vi "TEST - Convert Dirs to VI Libraries (proxy).vi"(8 "error in (no error)":errorcluster) -> (0 "error out":errorcluster, 2 "pass":bool)   [LabVIEW 2020]
uses:
  <userlib>/_OpenG.lib/error/error.llb/openg_error.lvlib
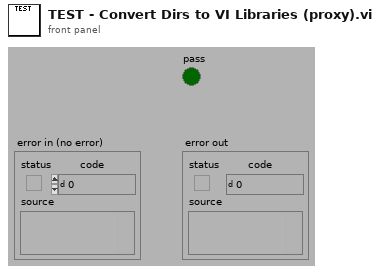
[diagram p1: front panel]
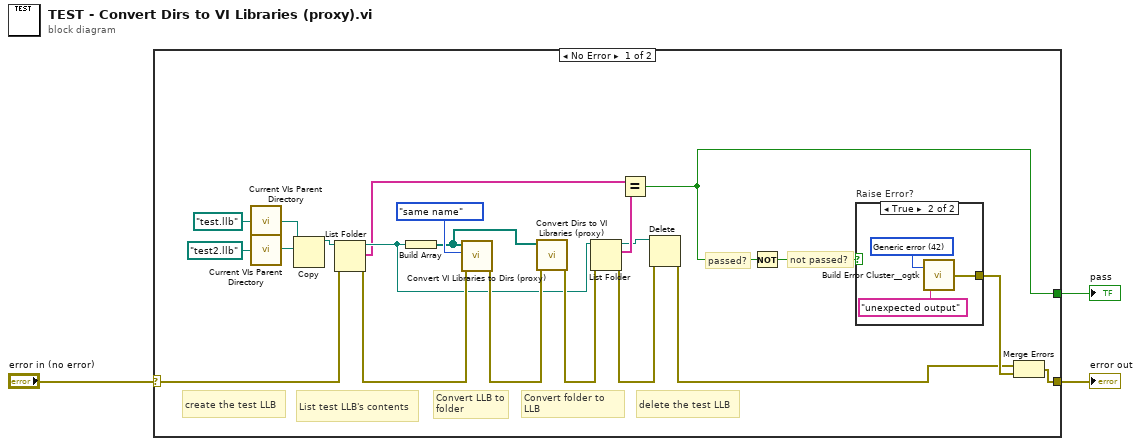
[diagram p0: block diagram]
diagram:
  n1 = case shown="No Error" "error in (no error)" {
    selector: "error in (no error)" -> [w15 w28]
    tunnel: [w5 _] -> w3
    tunnel: [w24 w28] -> w1
    frame No Error {
      # "create the test LLB"
      # "delete the test LLB"
      # "Convert folder to LLB"
      # "List test LLB's contents"
      # "Convert LLB to folder"
      # "not passed?"
      # "passed?"
      n2 = call "Current VIs Parent Directory.vi"("Relative path (.)"=path "test.llb") -> ("Parent Directory (+ Relative)"=w20:path)  [unwired: 4 in]
      n3 = call "Current VIs Parent Directory.vi"("Relative path (.)"=path "test2.llb") -> ("Parent Directory (+ Relative)"=w18:path)  [unwired: 4 in]
      n4 = Copy(10:w18, 11:w20) -> (3:w16:path)  [unwired: 3 in, 2 out]
      n5 = List Folder(path=w16, error in=w15) -> (path out=w8:path, filenames=w6:string[], error out=w14:errorcluster)  [unwired: 2 in, 1 out]
      n6 = Build Array(w8) -> (w12:path[])
      n7 = call "Convert VI Libraries to Dirs (proxy).vi"("error in (no error)"=w14, "dir name scheme (0:remove .llb)"=enum16{"remove .llb", "same name", "prompt"}."same name", "VI libraries"=w12) -> ("error out"=w11:errorcluster)  [unwired: 5 in, 3 out]
      n8 = call "Convert Dirs to VI Libraries (proxy).vi"("error in (no error)"=w11, "directories"=w12) -> ("error out"=w9:errorcluster)  [unwired: 9 in]
      n9 = List Folder(path=w8, error in=w9) -> (path out=w4:path, filenames=w7:string[], error out=w10:errorcluster)  [unwired: 2 in, 1 out]
      n10 = Equal?(x=w6, y=w7) -> (x = y?=w5:bool)
      n11 = Delete(path (use dialog)=w4, error in=w10) -> (error out=w17:errorcluster)  [unwired: 3 in, 2 out]
      n12 = Not(x=w5) -> (.not. x?=w22:bool)
      n13 = case "Raise Error?" shown="True" w22 {
        tunnel: [_ w25] -> w23
        frame False {
        }
        frame True {
          w26 = 42 items=["No error", "Argument error", "Memory is full", "Out of zone", "End of file", "File already open", "Generic file I/O error", "File not found", "File permission error", "Disk is full", "Duplicate path", "Too many files open", "System feature not enabled", "Resource file not found", "Cannot add resource", "Resource not found", "Image not found", "Image memory error", "Pen does not exist", "Config type invalid", "Config token not found", "Config parse error", "Config memory error", "Bad external code format", "Bad external code offset", "External code not present", "Null window", "Destroy window error", "Null menu", "Print aborted", "Bad print record", "Print driver error", "Windows error during printing", "Memory error during printing", "Print dialog error", "Generic print error", "Invalid device refnum", "Device not found", "Device parameter error", "Device unit error", "Cannot open device", "Device call aborted", "Generic error", "Cancelled by user", "Object ID too low", "Object ID too high", "Object not in heap", "Unknown heap", "Unknown object (invalid DefProc)", "Unknown object (DefProc not in table)", "Message out of range", "Invalid (null) method", "Unknown message", "Manager call not supported", "Bad address", "Network operation in progress", "Network operation timed out", "Connection is busy", "Network attribute not supported", "Network error", "Address in use", "System out of memory", "Connection aborted", "Connection refused", "Not connected", "Already connected", "Connection closed", "Initialization error (interapplication manager)", "Bad occurrence", "Wait on unbound occurrence handler", "Occurrence queue overflow", "Datalog type conflict", "Unused", "Unrecognized type (interapplication manager)", "Memory corrupt", "Failed to make temporary DLL", "Old CIN version", "Drag socket not found", "Failed to load drop-object", "Failed to register OLE object", "Failed to release OLE object", "Format specifier type mismatch", "Unknown format specifier", "Too few format specifiers", "Too many format specifiers", "Scan failed", "Newer CIN version", "Error converting to variant", "Runtime menu error", "Password tampered", "Variant attribute not found", "Incompatible variant data type", "Event data is not available", "Event Store is not present", "Occurrence is not found", "Event Queue is not created", "Event info is not available", "Refnum passed is NULL", "Error retrieving Class GUID", "Error retrieving CoClass GUID", "Error retrieving TypeLib GUID.", "Bad built application magic bytes.", "Specific driver is different from the specific driver associated with the Logical Name.", "There is no session opened to the class driver.", "Max Error", "MAX - Error with config objects", "MAX - Error loading configuration", "MAX - Group not supported"]
          n14 = call <userlib>:"Build Error Cluster__ogtk.vi"("String to Prepend to source (\"\")"="unexpected output" ("String to Prepend to source (\"\")"), "code"=w26) -> ("error out"=w25:errorcluster)
        }
      }
      n15 = Merge Errors(w17, w23) -> (w24:errorcluster)
    }
    frame Error {
    }
  }
  "pass" <- w3
  "error out" <- w1
